vi "From Variant.vi"(8 "error in (no error)":errorcluster, 10 "Variant":variant, 11 "Abs_Boolean_1D in":refnum<class "Abs_Boolean_1D.lvclass">) -> (0 "error out":errorcluster, 3 "Abs_Boolean_1D out":refnum<class "Abs_Boolean_1D.lvclass">)   [LabVIEW 2021, in "Abs_Boolean_1D.lvclass"]
uses:
  Abs_Boolean_1D.lvclass
  Support/Element Type.ctl
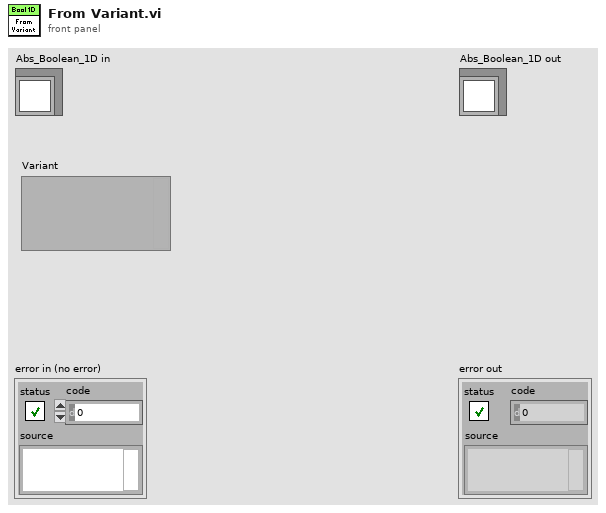
[diagram p1: front panel]
types:
  T1 = typedef "Abs_Boolean_1D.lvclass/Element Type.ctl" = bool
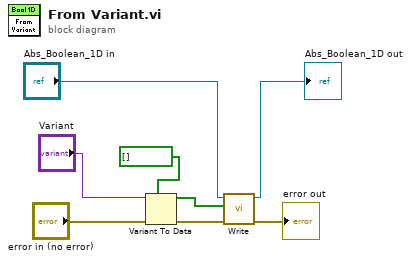
[diagram p0: block diagram]
diagram:
  n1 = Variant To Data(error in="error in (no error)", type=T1[] [] ("Boolean 1D"), Variant="Variant") -> (data=w3:T1[], error out=w6:errorcluster)
  n2 = call-dynamic "Write.vi"("error in (no error)"=w6, "Boolean 1D"=w3, "Boolean in"="Abs_Boolean_1D in") -> ("error out"=→"error out":errorcluster, "Boolean out"=→"Abs_Boolean_1D out":refnum<class "Abs_Boolean_1D.lvclass">)  [unwired: 7 in]
